vi "Parse.vi"(8 "error in (no error)":errorcluster, 10 "Data String":string, 11 "General Parser in":refnum<class "General Parser.lvclass">) -> (0 "error out":errorcluster, 2 "Data Values":dbl[](array[numeric]), 3 "General Parser out":refnum<class "General Parser.lvclass">)   [LabVIEW 2018, in "General Parser.lvclass"]
doc: "General Parser.lvclass:Parse.vi\n\nThis VI takes a string read from an instrument as input and returns an array of channel values.\n\nInstrument Communication Module Version 1.0\nSeptember, 2017 Original Code Consulting David Thomson\n www.originalcode.com"
uses:
  General Parser.lvclass
  General Parser.lvclass/General Parser.ctl
  ICM whitespace.ctl
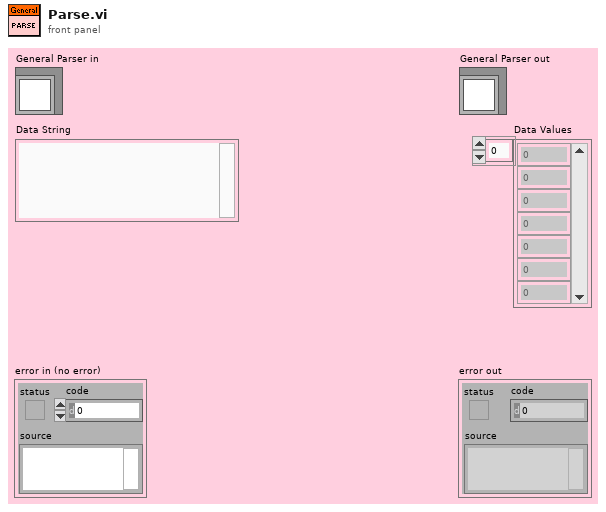
[diagram p1: front panel]
types:
  T1 = typedef "ICM whitespace.ctl" = u16
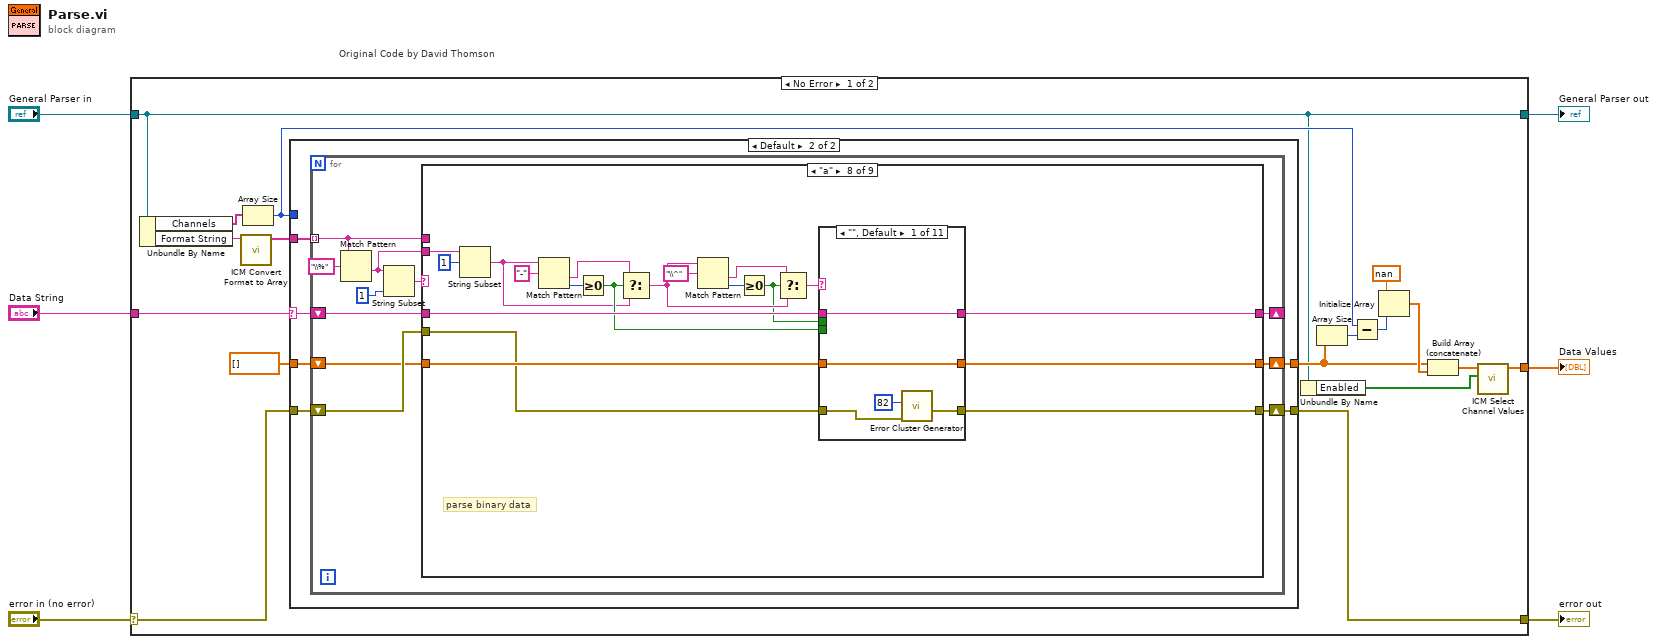
[diagram p0: block diagram]
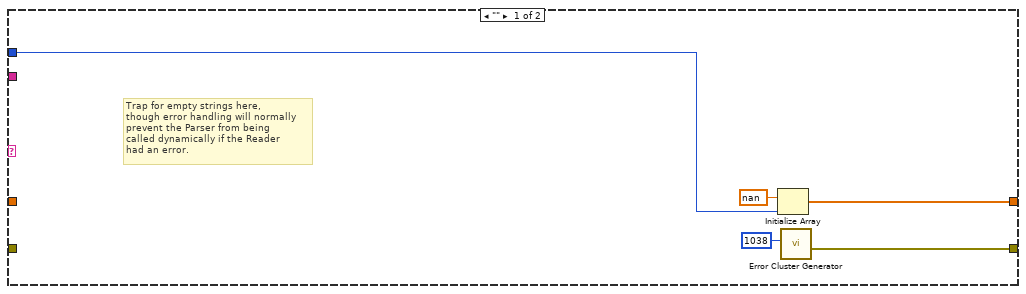
[diagram p2: hidden frame]
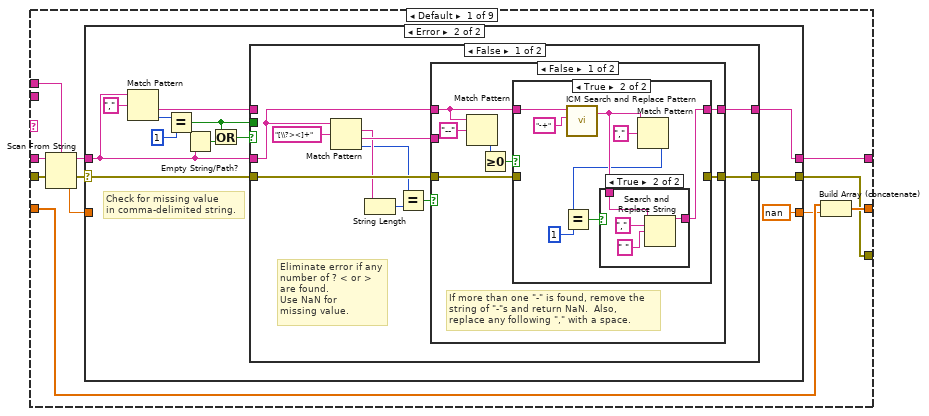
[diagram p3: hidden frame]
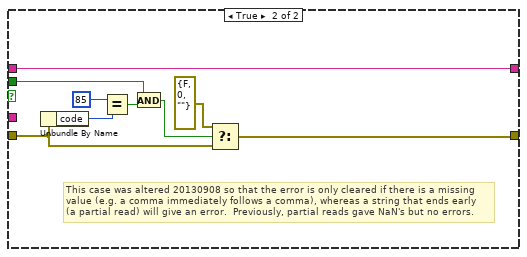
[diagram p8: hidden frame]
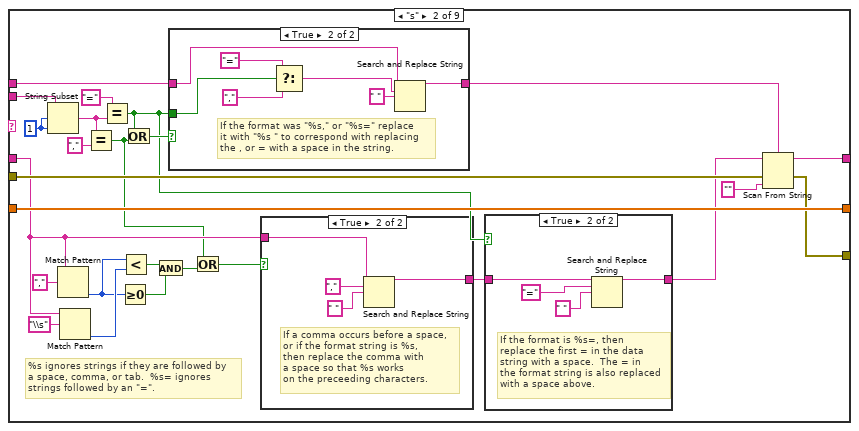
[diagram p9: hidden frame]
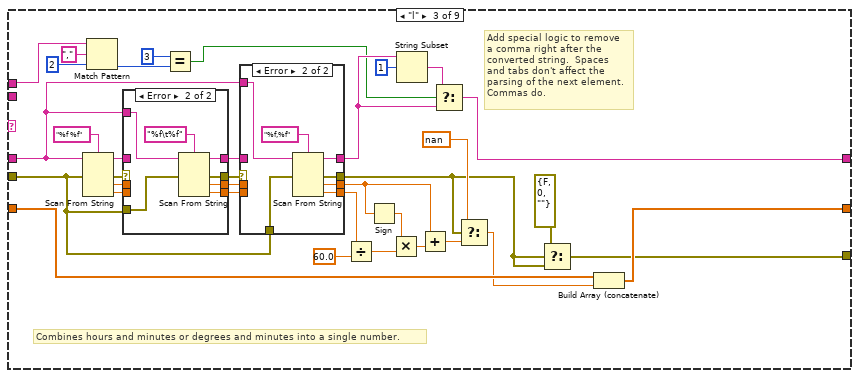
[diagram p13: hidden frame]
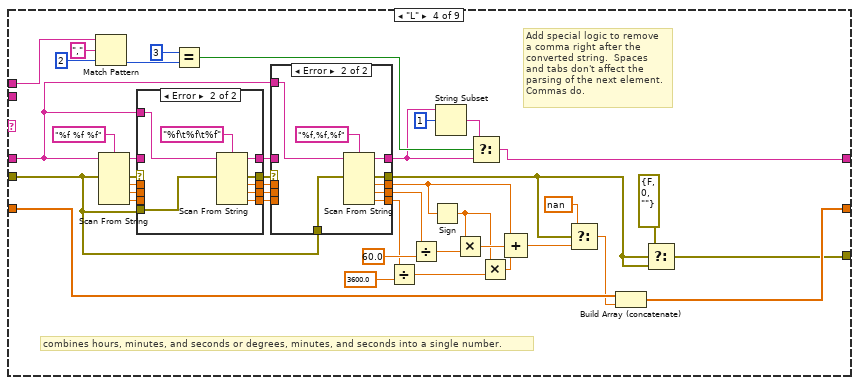
[diagram p16: hidden frame]
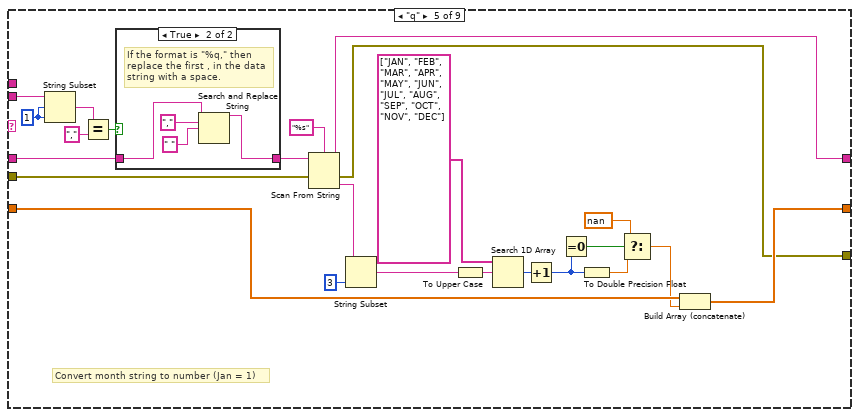
[diagram p19: hidden frame]
diagram:
  n1 = case "Original Code by David Thomson" shown="No Error" "error in (no error)" {
    selector: "error in (no error)" -> [w16 w569]
    tunnel: [w15 w569] -> w5
    tunnel: [w8 w568] -> w3
    tunnel: "General Parser in" -> [w8 w568]
    tunnel: "Data String" -> [w14 _]
    tunnel: [w9 _] -> w1
    frame No Error {
      n2 = Unbundle By Name(w8) -> ("Channels"=w12:string[], "Format String"=w13:string)
      n3 = call "ICM Convert Format to Array.vi"("Format String"=w13) -> ("Format Array"=w17:string[])  [unwired: 10 in]
      n4 = Array Size(array=w12) -> (size(s)=w11:i32)
      n5 = case shown="Default" w14 {
        selector: w14 -> [_ w29]
        tunnel: w16 -> [_ w34]
        tunnel: w17 -> [_ w33]
        tunnel: [w28 w32] -> w15
        tunnel: dbl[] [] ("Values") -> [_ w31]
        tunnel: [w25 w30] -> w18
        tunnel: w11 -> [w24 _]
        frame "" {
          # "Trap for empty strings here,\nthough error handling will normally\nprevent the Parser from being\ncalled dynamically if the Reader\nhad an error."
          n6 = Initialize Array(nan ("y"), w24) -> (w25:dbl[])
          n7 = call "Error Cluster Generator.vi"("code"=1038) -> ("error out"=w28:errorcluster)  [unwired: 5 in, 1 out]
        }
        frame Default {
          n8 = for {
            shift-right: [w38] -> _
            shift-left: w29 -> [w45]
            shift-right: [w39] -> w32
            shift-left: w34 -> [w44]
            tunnel: w33 -> [w36] mode=indexing
            shift-right: [w41] -> w30
            shift-left: w31 -> [w42]
            n9 = Match Pattern(string=w36, regular expression="\\%") -> (after substring=w35:string)  [unwired: 4 out]
            n10 = String Subset(string=w35, length (rest)=1 ("length (rest)")) -> (substring=w40:string)  [unwired: 1 out]
            n11 = case shown="\"a\"" w40 {
              selector: w40 -> [_ _ _ _ _ w322 _ _ _]
              tunnel: w45 -> [w56 w128 w175 w239 w283 w312 w417 w438 w529]
              tunnel: w44 -> [w55 w136 w174 w238 w301 w330 w415 w433 w532]
              tunnel: w36 -> [w54 w125 w170 w223 _ _ _ _ _]
              tunnel: [w53 w137 w186 w250 w299 w314 w418 w434 w530] -> w41
              tunnel: w42 -> [w48 w137 w187 w251 w300 _ w418 w435 w547]
              tunnel: [w51 w135 w158 w215 w297 w323 w415 w432 w533] -> w39
              tunnel: [w46 w139 w165 w219 w298 w324 w416 w437 w525] -> w38
              tunnel: w35 -> [_ w127 _ _ w285 _ w411 w431 w540]
              frame Default {
                n12 = Scan From String(format string=w54, input string=w56, error in=w55) -> (remaining string=w50:string, error out=w52:errorcluster, output 1=w49:dbl)  [unwired: 1 in, 2 out]
                n13 = case shown="Error" w52 {
                  selector: w52 -> [w59 w67]
                  tunnel: [w59 w61] -> w51
                  tunnel: [w58 w62] -> w46
                  tunnel: w50 -> [w58 w63]
                  tunnel: w49 -> [w57 _]
                  tunnel: [w57 nan ("y")] -> w47
                  frame No Error {
                    # "this case uses LabVIEW's built in parsing codes"
                  }
                  frame Error {
                    # "Check for missing value\nin comma-delimited string."
                    n14 = Match Pattern(string=w63, regular expression=",") -> (after substring=w68:string, offset past match=w70:i32)  [unwired: 3 out]
                    n15 = Equal?(x=w70, y=1) -> (x = y?=w60:bool)
                    n16 = Empty String/Path?(string/path=w63) -> (empty?=w64:bool)
                    n17 = Or(x=w60, y=w64) -> (x .or. y?=w65:bool)
                    n18 = case shown="False" w65 {
                      tunnel: [w77 w113] -> w62
                      tunnel: w68 -> [_ w113]
                      tunnel: w63 -> [w79 _]
                      tunnel: [w76 w112] -> w61
                      tunnel: w67 -> [w78 w111]
                      tunnel: w60 -> [_ w106]
                      frame False {
                        # "Eliminate error if any\nnumber of ? < or >\nare found.\nUse NaN for\nmissing value."
                        n19 = Match Pattern(string=w79, regular expression="[\\?><]+") -> (match substring=w74:string, after substring=w75:string, offset past match=w72:i32)  [unwired: 2 out]
                        n20 = String Length(string=w74) -> (length=w73:i32)
                        n21 = Equal?(x=w72, y=w73) -> (x = y?=w80:bool)
                        n22 = case shown="False" w80 {
                          tunnel: [w83 w104] -> w77
                          tunnel: w79 -> [w82 _]
                          tunnel: [w84 _] -> w76
                          tunnel: w78 -> [w85 _]
                          tunnel: w75 -> [_ w104]
                          frame False {
                            # "If more than one \"-\" is found, remove the\nstring of \"-\"s and return NaN.  Also,\nreplace any following \",\" with a space."
                            n23 = Match Pattern(string=w82, regular expression="--") -> (offset past match=w87:i32)  [unwired: 4 out]
                            n24 = Greater Or Equal To 0?(x=w87) -> (x >= 0?=w86:bool)
                            n25 = case shown="True" w86 {
                              tunnel: [w90 _] -> w84
                              tunnel: w85 -> [w90 _]
                              tunnel: [w89 w96] -> w83
                              tunnel: w82 -> [w89 w98]
                              frame False {
                              }
                              frame True {
                                n26 = call "ICM Search and Replace Pattern.vi"("string"=w98, "regular expression (\"\")"="-+" ("regular expression (\"\")")) -> ("result string"=w94:string)  [unwired: 1 in, 3 out]
                                n27 = Match Pattern(string=w94, regular expression=",") -> (offset past match=w92:i32)  [unwired: 4 out]
                                n28 = Equal?(x=w92, y=1) -> (x = y?=w91:bool)
                                n29 = case shown="True" w91 {
                                tunnel: w94 -> [w99 w101]
                                tunnel: [w99 w100] -> w96
                                frame False {
                                }
                                frame True {
                                n30 = Search and Replace String(input string=w101, search string=",", replace string=" " ("replace string (\"\")")) -> (result string=w100:string)  [unwired: 1 in, 7 out]
                                }
                                }
                              }
                            }
                          }
                          frame True {
                          }
                        }
                      }
                      frame True {
                        # "This case was altered 20130908 so that the error is only cleared if there is a missing\nvalue (e.g. a comma immediately follows a comma), whereas a string that ends early\n(a partial read) will give an error.  Previously, partial reads gave NaN's but no errors."
                        n31 = Unbundle By Name(w111) -> ("code"=w110:i32)
                        n32 = Equal?(x=85, y=w110) -> (x = y?=w107:bool)
                        n33 = And(x=w106, y=w107) -> (x .and. y?=w105:bool)
                        n34 = Select(t=errorcluster {"status"=FALSE, "code"=0, "source"=""}, s=w105, f=w111) -> (s? t:f=w112:errorcluster)
                      }
                    }
                  }
                }
                n35 = Build Array (concatenate)(w48, w47) -> (w53:dbl[])
              }
              frame "s" {
                w123 = 1 ("length (rest)")
                # "%s ignores strings if they are followed by\na space, comma, or tab.  %s= ignores\nstrings followed by an \"=\"."
                n36 = String Subset(string=w127, offset (0)=w123, length (rest)=w123) -> (substring=w121:string)
                n37 = Match Pattern(string=w128, regular expression=",") -> (offset past match=w130:i32)  [unwired: 4 out]
                n38 = Match Pattern(string=w128, regular expression="\\s") -> (offset past match=w132:i32)  [unwired: 4 out]
                n39 = Equal?(x=w121, y=",") -> (x = y?=w115:bool)
                n40 = Equal?(x="=" ("y"), y=w121) -> (x = y?=w117:bool)
                n41 = Greater Or Equal To 0?(x=w130) -> (x >= 0?=w129:bool)
                n42 = Less?(x=w130, y=w132) -> (x < y?=w131:bool)
                n43 = Or(x=w117, y=w115) -> (x .or. y?=w122:bool)
                n44 = And(x=w131, y=w129) -> (x .and. y?=w116:bool)
                n45 = case shown="True" w122 {
                  tunnel: [w145 w150] -> w124
                  tunnel: w125 -> [w145 w151]
                  tunnel: w117 -> [_ w146]
                  frame False {
                  }
                  frame True {
                    # "If the format was \"%s,\" or \"%s=\" replace\nit with \"%s \" to correspond with replacing\nthe , or = with a space in the string."
                    n46 = Select(t="=" ("y"), s=w146, f="," ("search string")) -> (s? t:f=w147:string)
                    n47 = Search and Replace String(input string=w151, search string=w147, replace string=" " ("replace string (\"\")")) -> (result string=w150:string)  [unwired: 1 in, 7 out]
                  }
                }
                n48 = Or(x=w115, y=w116) -> (x .or. y?=w114:bool)
                n49 = case shown="True" w114 {
                  tunnel: [w153 w155] -> w119
                  tunnel: w128 -> [w153 w154]
                  frame False {
                  }
                  frame True {
                    # "If a comma occurs before a space, \nor if the format string is %s,\nthen replace the comma with\na space so that %s works\non the preceeding characters."
                    n50 = Search and Replace String(input string=w154, search string=",", replace string=" " ("replace string (\"\")")) -> (result string=w155:string)  [unwired: 1 in, 7 out]
                  }
                }
                n51 = case shown="True" w117 {
                  tunnel: w119 -> [w140 w142]
                  tunnel: [w140 w141] -> w118
                  frame False {
                  }
                  frame True {
                    # "If the format is %s=, then\nreplace the first = in the data\nstring with a space.  The = in\nthe format string is also replaced\nwith a space above."
                    n52 = Search and Replace String(input string=w142, search string="=", replace string=" " ("replace string (\"\")")) -> (result string=w141:string)  [unwired: 1 in, 7 out]
                  }
                }
                n53 = Scan From String(format string=w124, input string=w118, error in=w136, default 1="") -> (remaining string=w139:string, error out=w135:errorcluster)  [unwired: 1 in, 2 out]
              }
              frame "l" {
                # "Combines hours and minutes or degrees and minutes into a single number."
                # "Add special logic to remove\na comma right after the\nconverted string.  Spaces\nand tabs don't affect the\nparsing of the next element.\nCommas do."
                n54 = Scan From String(format string="%f %f", input string=w175, error in=w174) -> (remaining string=w182:string, error out=w185:errorcluster, output 1=w184:dbl, output 2=w183:dbl)  [unwired: 1 in, 3 out]
                n55 = Match Pattern(string=w170, regular expression=",", offset (0)=2) -> (offset past match=w163:i32)  [unwired: 3 out]
                n56 = case shown="Error" w185 {
                  selector: w185 -> [w207 _]
                  tunnel: [w207 w208] -> w181
                  tunnel: [w206 w213] -> w180
                  tunnel: w184 -> [w206 _]
                  tunnel: [w205 w212] -> w179
                  tunnel: w183 -> [w205 _]
                  tunnel: w182 -> [w204 _]
                  tunnel: [w204 w211] -> w176
                  tunnel: w175 -> [_ w210]
                  tunnel: w174 -> [_ w209]
                  frame No Error {
                  }
                  frame Error {
                    n57 = Scan From String(format string="%f\t%f", input string=w210, error in=w209) -> (remaining string=w211:string, error out=w208:errorcluster, output 1=w213:dbl, output 2=w212:dbl)  [unwired: 1 in, 3 out]
                  }
                }
                n58 = Equal?(x=3, y=w163) -> (x = y?=w162:bool)
                n59 = case shown="Error" w181 {
                  selector: w181 -> [w196 _]
                  tunnel: [w196 w200] -> w159
                  tunnel: [w195 w202] -> w178
                  tunnel: w180 -> [w195 _]
                  tunnel: [w194 w201] -> w177
                  tunnel: w179 -> [w194 _]
                  tunnel: w176 -> [w193 _]
                  tunnel: [w193 w199] -> w164
                  tunnel: w175 -> [_ w198]
                  tunnel: w174 -> [_ w197]
                  frame No Error {
                  }
                  frame Error {
                    n60 = Scan From String(format string="%f,%f", input string=w198, error in=w197) -> (remaining string=w199:string, error out=w200:errorcluster, output 1=w202:dbl, output 2=w201:dbl)  [unwired: 1 in, 3 out]
                  }
                }
                n61 = Divide(x=w177, y=60.0) -> (x/y=w190:dbl)
                n62 = Sign(1:w178) -> (0:w189:dbl)
                n63 = Multiply(x=w189, y=w190) -> (x*y=w188:dbl)
                n64 = String Subset(string=w164, offset (0)=1) -> (substring=w166:string)  [unwired: 1 out]
                n65 = Add(x=w178, y=w188) -> (x+y=w173:dbl)
                n66 = Select(t=w166, s=w162, f=w164) -> (s? t:f=w165:string)
                n67 = Select(t=nan ("y"), s=w159, f=w173) -> (s? t:f=w172:dbl)
                n68 = Select(t=errorcluster {"status"=FALSE, "code"=0, "source"=""}, s=w159, f=w159) -> (s? t:f=w158:errorcluster)
                n69 = Build Array (concatenate)(w187, w172) -> (w186:dbl[])
              }
              frame "L" {
                # "combines hours, minutes, and seconds or degrees, minutes, and seconds into a single number."
                # "Add special logic to remove\na comma right after the\nconverted string.  Spaces\nand tabs don't affect the\nparsing of the next element.\nCommas do."
                n70 = Match Pattern(string=w223, regular expression=",", offset (0)=2) -> (offset past match=w225:i32)  [unwired: 3 out]
                n71 = Scan From String(format string="%f %f %f", input string=w239, error in=w238) -> (remaining string=w246:string, error out=w249:errorcluster, output 1=w248:dbl, output 2=w247:dbl, output 3=w234:dbl)  [unwired: 1 in, 4 out]
                n72 = case shown="Error" w249 {
                  selector: w249 -> [w273 _]
                  tunnel: [w273 w275] -> w245
                  tunnel: [w272 w280] -> w244
                  tunnel: w248 -> [w272 _]
                  tunnel: [w271 w279] -> w243
                  tunnel: w247 -> [w271 _]
                  tunnel: w246 -> [w270 _]
                  tunnel: [w270 w278] -> w240
                  tunnel: w239 -> [_ w277]
                  tunnel: w238 -> [_ w276]
                  tunnel: w234 -> [w269 _]
                  tunnel: [w269 w274] -> w233
                  frame No Error {
                  }
                  frame Error {
                    n73 = Scan From String(format string="%f\t%f\t%f", input string=w277, error in=w276) -> (remaining string=w278:string, error out=w275:errorcluster, output 1=w280:dbl, output 2=w279:dbl, output 3=w274:dbl)  [unwired: 1 in, 4 out]
                  }
                }
                n74 = Equal?(x=3, y=w225) -> (x = y?=w220:bool)
                n75 = case shown="Error" w245 {
                  selector: w245 -> [w260 _]
                  tunnel: [w260 w265] -> w216
                  tunnel: [w259 w267] -> w242
                  tunnel: w244 -> [w259 _]
                  tunnel: [w258 w266] -> w241
                  tunnel: w243 -> [w258 _]
                  tunnel: w240 -> [w257 _]
                  tunnel: [w257 w264] -> w218
                  tunnel: w239 -> [_ w263]
                  tunnel: w238 -> [_ w262]
                  tunnel: [w256 w261] -> w230
                  tunnel: w233 -> [w256 _]
                  frame No Error {
                  }
                  frame Error {
                    n76 = Scan From String(format string="%f,%f,%f", input string=w263, error in=w262) -> (remaining string=w264:string, error out=w265:errorcluster, output 1=w267:dbl, output 2=w266:dbl, output 3=w261:dbl)  [unwired: 1 in, 4 out]
                  }
                }
                n77 = Divide(x=w230, y=3600.0) -> (x/y=w232:dbl)
                n78 = Divide(x=w241, y=60.0) -> (x/y=w253:dbl)
                n79 = Sign(1:w242) -> (0:w229:dbl)
                n80 = String Subset(string=w218, offset (0)=1) -> (substring=w221:string)  [unwired: 1 out]
                n81 = Multiply(x=w229, y=w253) -> (x*y=w252:dbl)
                n82 = Select(t=w221, s=w220, f=w218) -> (s? t:f=w219:string)
                n83 = Multiply(x=w229, y=w232) -> (x*y=w228:dbl)
                n84 = Compound Arithmetic op=ADD(w242, w252, w228) -> (w237:dbl)
                n85 = Select(t=nan ("y"), s=w216, f=w237) -> (s? t:f=w236:dbl)
                n86 = Build Array (concatenate)(w251, w236) -> (w250:dbl[])
                n87 = Select(t=errorcluster {"status"=FALSE, "code"=0, "source"=""}, s=w216, f=w216) -> (s? t:f=w215:errorcluster)
              }
              frame "q" {
                w287 = 1 ("length (rest)")
                # "Convert month string to number (Jan = 1)"
                n88 = String Subset(string=w285, offset (0)=w287, length (rest)=w287) -> (substring=w286:string)
                n89 = Equal?(x=w286, y=",") -> (x = y?=w284:bool)
                n90 = case shown="True" w284 {
                  tunnel: w283 -> [w306 w308]
                  tunnel: [w306 w307] -> w282
                  frame False {
                  }
                  frame True {
                    # "If the format is \"%q,\" then\nreplace the first , in the data\nstring with a space."
                    n91 = Search and Replace String(input string=w308, search string=",", replace string=" " ("replace string (\"\")")) -> (result string=w307:string)  [unwired: 1 in, 7 out]
                  }
                }
                n92 = Scan From String(format string="%s", input string=w282, error in=w301) -> (remaining string=w298:string, error out=w297:errorcluster, output 1=w296:string)  [unwired: 1 in, 2 out]
                n93 = String Subset(string=w296, length (rest)=3 ("length (rest)")) -> (substring=w294:string)  [unwired: 1 out]
                n94 = To Upper Case(1:w294) -> (0:w303:string)
                n95 = Search 1D Array(1D array=string[] ["JAN", "FEB", "MAR", "APR", "MAY", "JUN", "JUL", "AUG", "SEP", "OCT", "NOV", "DEC"], element=w303) -> (index of element=w305:i32)  [unwired: 1 out]
                n96 = Increment(x=w305) -> (x+1=w293:i32)
                n97 = Equal To 0?(x=w293) -> (x = 0?=w292:bool)
                n98 = To Double Precision Float(number=w293) -> (double precision float=w291:dbl)
                n99 = Select(t=nan ("y"), s=w292, f=w291) -> (s? t:f=w290:dbl)
                n100 = Build Array (concatenate)(w300, w290) -> (w299:dbl[])
              }
              frame "I", "i" {
                w311 = T1 1 items=["both", "start of string", "end of string"] ("location (both)")
                # "decodes ISO 8601 time strings\n\"I\" includes a time stamp before\nthe other channels"
                n101 = call "ICM Trim Whitespace.vi"("string"=w312, "location (both)"=w311) -> ("trimmed string"=w313:string)
                n102 = Match Pattern(string=w313, regular expression="[T\\s]") -> (before substring=w331:string, after substring=w326:string)  [unwired: 3 out]
                n103 = Match Pattern(string=w326, regular expression="[\\s\\t,]") -> (before substring=w325:string, after substring=w324:string)  [unwired: 3 out]
                n104 = Match Pattern(string=w331, regular expression="-") -> (offset past match=w332:i32)  [unwired: 4 out]
                n105 = case "Decode Date" shown="5" w332 {
                  tunnel: w331 -> [w390 w403]
                  tunnel: [w387 w400] -> w316
                  tunnel: [w382 w399] -> w315
                  tunnel: [w388 w401] -> w317
                  tunnel: w330 -> [w381 w397]
                  tunnel: [w378 w396] -> w318
                  frame 0, Default {
                    w384 = 0.0 ("default value 1")
                    w383 = "%d" ("format string")
                    n106 = String Subset(string=w390, length (rest)=4 ("length (rest)")) -> (substring=w389:string)  [unwired: 1 out]
                    n107 = String Subset(string=w390, offset (0)=4, length (rest)=2 ("length (rest)")) -> (substring=w386:string)
                    n108 = String Subset(string=w390, offset (0)=6, length (rest)=2 ("length (rest)")) -> (substring=w385:string)
                    n109 = Scan From String(format string=w383, input string=w385, error in=w381, default 1=w384) -> (error out=w380:errorcluster, output 1=w382:dbl)  [unwired: 1 in, 2 out]
                    n110 = Scan From String(format string=w383, input string=w386, error in=w380, default 1=w384) -> (error out=w379:errorcluster, output 1=w387:dbl)  [unwired: 1 in, 2 out]
                    n111 = Scan From String(format string=w383, input string=w389, error in=w379, default 1=w384) -> (error out=w378:errorcluster, output 1=w388:dbl)  [unwired: 1 in, 2 out]
                  }
                  frame 5 {
                    w398 = 0.0 ("default value 1")
                    n112 = Scan From String(format string="%d-%d-%d", input string=w403, error in=w397, default 1=w398, default 2=w398, default 3=w398) -> (error out=w396:errorcluster, output 1=w401:dbl, output 2=w400:dbl, output 3=w399:dbl)  [unwired: 1 in, 2 out]
                  }
                }
                n113 = Match Pattern(string=w325, regular expression=":") -> (offset past match=w328:i32)  [unwired: 4 out]
                n114 = case "Decode Time" shown="3" w328 {
                  tunnel: w325 -> [w364 w377]
                  tunnel: [w362 w374] -> w320
                  tunnel: [w357 w373] -> w319
                  tunnel: [w351 w375] -> w321
                  tunnel: w318 -> [w356 w371]
                  tunnel: [w353 w370] -> w323
                  frame 0, Default {
                    w359 = 0.0 ("default value 1")
                    w358 = "%d" ("format string")
                    n115 = String Subset(string=w364, length (rest)=2 ("length (rest)")) -> (substring=w363:string)  [unwired: 1 out]
                    n116 = String Subset(string=w364, offset (0)=2, length (rest)=2 ("length (rest)")) -> (substring=w361:string)
                    n117 = String Subset(string=w364, offset (0)=4, length (rest)=2 ("length (rest)")) -> (substring=w360:string)
                    n118 = Scan From String(format string="%f", input string=w360, error in=w356, default 1=w359) -> (error out=w355:errorcluster, output 1=w357:dbl)  [unwired: 1 in, 2 out]
                    n119 = Scan From String(format string=w358, input string=w361, error in=w355, default 1=w359) -> (error out=w354:errorcluster, output 1=w362:dbl)  [unwired: 1 in, 2 out]
                    n120 = Scan From String(format string=w358, input string=w363, error in=w354, default 1=w359) -> (error out=w353:errorcluster, output 1=w351:dbl)  [unwired: 1 in, 2 out]
                  }
                  frame 3 {
                    w372 = 0.0 ("default value 1")
                    n121 = Scan From String(format string="%d:%d:%f", input string=w377, error in=w371, default 1=w372, default 2=w372, default 3=w372) -> (error out=w370:errorcluster, output 1=w375:dbl, output 2=w374:dbl, output 3=w373:dbl)  [unwired: 1 in, 2 out]
                  }
                }
                n122 = case shown="\"I\"" w322 {
                  tunnel: w321 -> [w338 w350]
                  tunnel: w320 -> [w337 w345]
                  tunnel: w319 -> [w336 w346]
                  tunnel: w317 -> [w341 w342]
                  tunnel: w316 -> [w340 w343]
                  tunnel: w315 -> [w339 w344]
                  tunnel: [w335 w349] -> w314
                  frame "i", Default {
                    n123 = Build Array(w341, w340, w339, w338, w337, w336) -> (w335:dbl[])
                  }
                  frame "I" {
                    n124 = call "ICM Calculate Time Stamps.vi"("Second"=w346, "Year"=w342, "Minute"=w345, "Hour"=w345, "Day"=w344, "Month"=w343) -> ("Seconds Since Midnight"=w348:dbl, "TimeStamp"=w347:dbl)  [unwired: 4 in]
                    n125 = Build Array(w347, w348, w342, w343, w344, w350, w345, w346) -> (w349:dbl[])
                  }
                }
              }
              frame "z" {
                w408 = "," ("regular expression")
                # "special case for %z with no \"n\" following it - skip one character"
                # "%zn ignores n characters"
                n126 = Match Pattern(string=w411, regular expression=w408) -> (before substring=w410:string, match substring=w409:string)  [unwired: 3 out]
                n127 = Equal?(x=w409, y=w408) -> (x = y?=w406:bool)
                n128 = String Length(string=w410) -> (length=w413:i32)
                n129 = Greater?(x=w413, y=1) -> (0:w414:bool)
                n130 = case shown="True" w414 {
                  tunnel: w410 -> [_ w422]
                  tunnel: [1 w420] -> w405
                  frame False {
                  }
                  frame True {
                    n131 = Scan From String(format string="z%d", input string=w422) -> (output 1=w420:i32)  [unwired: 2 in, 4 out]
                  }
                }
                n132 = Increment(x=w405) -> (x+1=w404:i32)
                n133 = Select(t=w404, s=w406, f=w405) -> (s? t:f=w407:i32)
                n134 = String Subset(string=w417, offset (0)=w407) -> (substring=w416:string)  [unwired: 1 out]
              }
              frame "a" {
                # "parse binary data"
                n135 = String Subset(string=w431, offset (0)=1) -> (substring=w430:string)  [unwired: 1 out]
                n136 = Match Pattern(string=w430, regular expression="-") -> (after substring=w439:string, offset past match=w440:i32)  [unwired: 3 out]
                n137 = Greater Or Equal To 0?(x=w440) -> (x >= 0?=w436:bool)
                n138 = Select(t=w439, s=w436, f=w430) -> (s? t:f=w424:string)
                n139 = Match Pattern(string=w424, regular expression="\\^") -> (after substring=w427:string, offset past match=w425:i32)  [unwired: 3 out]
                n140 = Greater Or Equal To 0?(x=w425) -> (x >= 0?=w423:bool)
                n141 = Select(t=w427, s=w423, f=w424) -> (s? t:f=w426:string)
                n142 = case shown="\"\", Default" w426 {
                  tunnel: w438 -> [w446 w452 w461 w469 w477 w483 w492 w500 w508 w516 w524]
                  tunnel: [w446 w451 w460 w468 w476 w482 w491 w499 w507 w515 w523] -> w437
                  tunnel: w436 -> [_ _ w455 w467 w475 _ w486 w498 w506 w514 w522]
                  tunnel: w435 -> [w445 w450 w459 w466 w474 w481 w490 w497 w505 w513 w521]
                  tunnel: [w445 w448 w457 w464 w472 w479 w488 w495 w503 w511 w519] -> w434
                  tunnel: [w444 w447 w456 w463 w471 w478 w487 w494 w502 w510 w518] -> w432
                  tunnel: w433 -> [w443 w447 w456 w463 w471 w478 w487 w494 w502 w510 w518]
                  tunnel: w423 -> [_ _ w454 w462 w470 _ w485 w493 w501 w509 w517]
                  frame "", Default {
                    n143 = call "Error Cluster Generator.vi"("error in"=w443, "code"=82) -> ("error out"=w444:errorcluster)  [unwired: 4 in, 1 out]
                  }
                  frame "U8" {
                    n144 = call "ICM aU8.vi"("String In"=w452) -> ("Value"=w449:dbl, "String Out"=w451:string)  [unwired: 1 in, 8 out]
                    n145 = Build Array (concatenate)(w450, w449) -> (w448:dbl[])
                  }
                  frame "U16" {
                    n146 = Or(x=w454, y=w455) -> (x .or. y?=w453:bool)
                    n147 = call "ICM aU16.vi"("Reverse Bytes"=w453, "String In"=w461) -> ("Value"=w458:dbl, "String Out"=w460:string)  [unwired: 8 out]
                    n148 = Build Array (concatenate)(w459, w458) -> (w457:dbl[])
                  }
                  frame "U32" {
                    n149 = call "ICM aU32.vi"("Reverse Bytes"=w467, "Swap Bytes"=w462, "String In"=w469) -> ("Value"=w465:dbl, "String Out"=w468:string)  [unwired: 1 in, 6 out]
                    n150 = Build Array (concatenate)(w466, w465) -> (w464:dbl[])
                  }
                  frame "U64" {
                    n151 = call "ICM aU64.vi"("Reverse Bytes"=w475, "Swap Bytes"=w470, "String In"=w477) -> ("Value"=w473:dbl, "String Out"=w476:string)  [unwired: 7 out]
                    n152 = Build Array (concatenate)(w474, w473) -> (w472:dbl[])
                  }
                  frame "I8" {
                    n153 = call "ICM aI8.vi"("String In"=w483) -> ("Value"=w480:dbl, "String Out"=w482:string)  [unwired: 1 in, 8 out]
                    n154 = Build Array (concatenate)(w481, w480) -> (w479:dbl[])
                  }
                  frame "I16" {
                    n155 = Or(x=w485, y=w486) -> (x .or. y?=w484:bool)
                    n156 = call "ICM aI16.vi"("Swap Bytes"=w484, "String In"=w492) -> ("Value"=w489:dbl, "String Out"=w491:string)  [unwired: 8 out]
                    n157 = Build Array (concatenate)(w490, w489) -> (w488:dbl[])
                  }
                  frame "I32" {
                    n158 = call "ICM aI32.vi"("Reverse Bytes"=w498, "Swap Bytes"=w493, "String In"=w500) -> ("Value"=w496:dbl, "String Out"=w499:string)  [unwired: 7 out]
                    n159 = Build Array (concatenate)(w497, w496) -> (w495:dbl[])
                  }
                  frame "I64" {
                    n160 = call "ICM aI64.vi"("Reverse Bytes"=w506, "Swap Bytes"=w501, "String In"=w508) -> ("Value"=w504:dbl, "String Out"=w507:string)  [unwired: 7 out]
                    n161 = Build Array (concatenate)(w505, w504) -> (w503:dbl[])
                  }
                  frame "SGL" {
                    n162 = call "ICM aSGL.vi"("Reverse Bytes"=w514, "Swap Bytes"=w509, "String In"=w516) -> ("Value"=w512:dbl, "String Out"=w515:string)  [unwired: 7 out]
                    n163 = Build Array (concatenate)(w513, w512) -> (w511:dbl[])
                  }
                  frame "DBL" {
                    n164 = call "ICM aDBL.vi"("Reverse Bytes"=w522, "Swap Bytes"=w517, "String In"=w524) -> ("Value"=w520:dbl, "String Out"=w523:string)  [unwired: 7 out]
                    n165 = Build Array (concatenate)(w521, w520) -> (w519:dbl[])
                  }
                }
              }
              frame "c" {
                # "scale the previous channel by a polynomial"
                n166 = Delete From Array(array=w547) -> (deleted portion=w527:dbl, array with subset deleted=w531:dbl[])  [unwired: 2 in]
                n167 = Match Pattern(string=w540, regular expression="\\[", offset (0)=1) -> (after substring=w546:string, offset past match=w538:i32)  [unwired: 2 out]
                n168 = Match Pattern(string=w546, regular expression="\\]") -> (before substring=w544:string, offset past match=w536:i32)  [unwired: 3 out]
                n169 = Spreadsheet String To Array(delimiter (Tab)=",", format string="%f", spreadsheet string=w544, array type (2D Dbl)=dbl[] []) -> (array=w528:dbl[])
                n170 = Less Than 0?(x=w538) -> (x < 0?=w537:bool)
                n171 = Less Than 0?(x=w536) -> (x < 0?=w535:bool)
                n172 = Or(x=w537, y=w535) -> (x .or. y?=w534:bool)
                n173 = case shown="False" w534 {
                  tunnel: [w555 w566] -> w533
                  tunnel: w532 -> [w555 w565]
                  tunnel: [w554 w564] -> w530
                  tunnel: w531 -> [w553 w564]
                  tunnel: w529 -> [w552 w563]
                  tunnel: [w552 w563] -> w525
                  tunnel: w528 -> [w551 _]
                  tunnel: w527 -> [w550 _]
                  frame False {
                    n174 = for {
                      tunnel: w551 -> [w562] mode=indexing
                      tunnel: w550 -> [w558]
                      shift-right: [w561] -> w548
                      shift-left: 0.0 ("Numeric") -> [w559]
                      i -> [w557]
                      n175 = Power Of X(1:w558, 2:w557) -> (0:w556:dbl)
                      n176 = Multiply(x=w562, y=w556) -> (x*y=w560:dbl)
                      n177 = Add(x=w560, y=w559) -> (x+y=w561:dbl)
                    }
                    n178 = Build Array (concatenate)(w553, w548) -> (w554:dbl[])
                  }
                  frame True {
                    n179 = call "Error Cluster Generator.vi"("error in"=w565, "code"=82) -> ("error out"=w566:errorcluster)  [unwired: 2 in, 3 out]
                  }
                }
              }
            }
          }
        }
      }
      n180 = Unbundle By Name(w8) -> ("Enabled"=w7:bool[])
      n181 = Array Size(array=w18) -> (size(s)=w21:i32)
      n182 = Subtract(x=w11, y=w21) -> (x-y=w20:i32)
      n183 = Initialize Array(nan ("y"), w20) -> (w19:dbl[])
      n184 = Build Array (concatenate)(w18, w19) -> (w10:dbl[])
      n185 = call "ICM Select Channel Values.vi"("Enabled"=w7, "Channel Values"=w10) -> ("Enabled Values"=w9:dbl[])  [unwired: 9 in]
    }
    frame Error {
    }
  }
  "error out" <- w5
  "General Parser out" <- w3
  "Data Values" <- w1
